vi "setup file.vi"(4 "frame rate":dbl, 5 "accel range":dbl, 6 "counts per rev":dbl, 7 "gyro range":dbl, 8 "error in (no error)":errorcluster, 11 "selected path":path) -> (0 "error out":errorcluster, 1 "channel names":string[](array[string]), 3 "tdms file out":refnum<k34>)   [LabVIEW 2012]
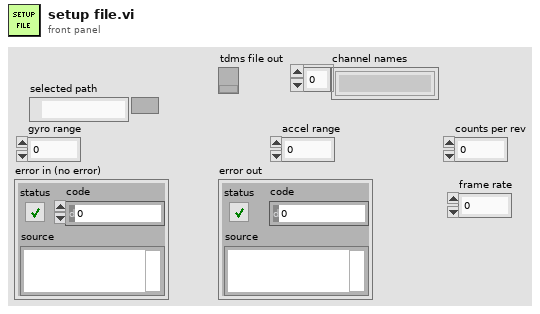
[diagram p1: front panel]
types:
  T1 = enum16{"open", "open or create", "create or replace", "create", "open (read-only)"}
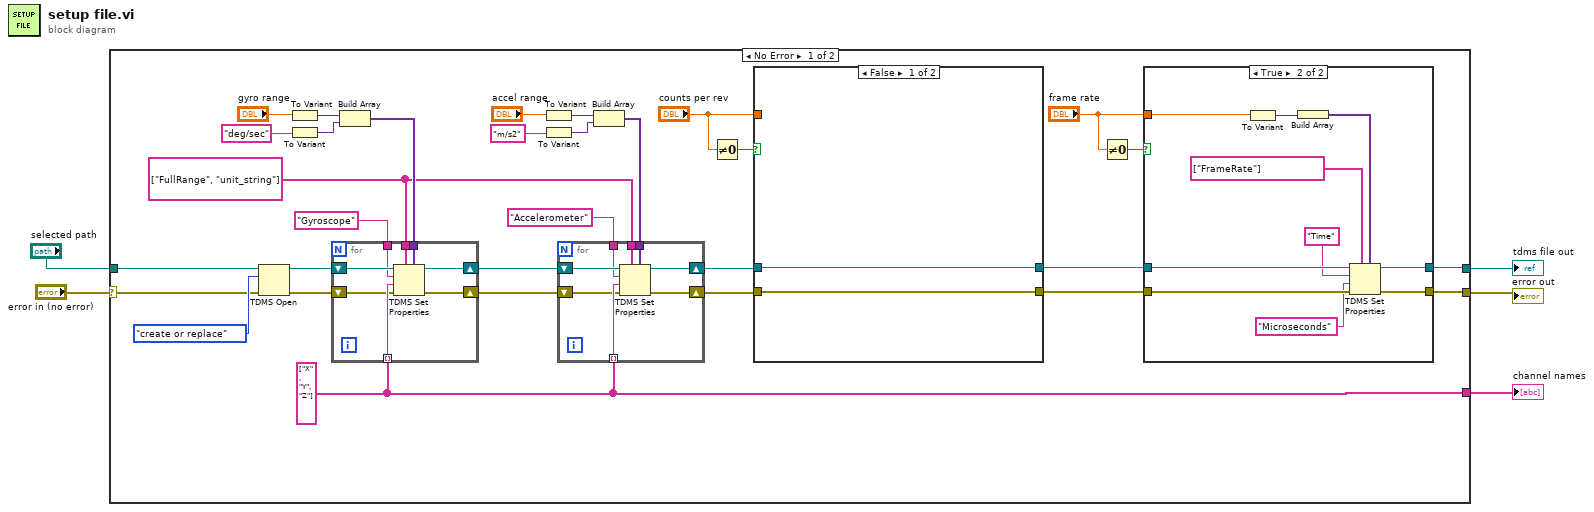
[diagram p0: block diagram]
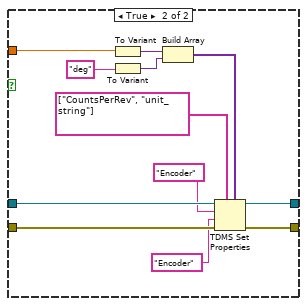
[diagram p3: hidden frame]
diagram:
  n1 = case shown="No Error" "error in (no error)" {
    selector: "error in (no error)" -> [w17 w79]
    tunnel: "selected path" -> [w35 _]
    tunnel: [w7 _] -> w3
    tunnel: [w6 w79] -> w2
    tunnel: [w16 _] -> w1
    frame No Error {
      w23 = string[] ["FullRange", "unit_string"] ("property names")
      w16 = string[] ["X", "Y", "Z"] ("channel name(s)")
      n2 = TDMS Open(8:w17, 10:T1."create or replace" ("operation (0:open)"), 11:w35) -> (0:w32:errorcluster, 3:w34:refnum<k34>)  [unwired: 3 in]
      n3 = To Variant(anything="gyro range") -> (Variant=w29:variant)
      n4 = To Variant(anything="deg/sec" ("group name (Untitled)")) -> (Variant=w28:variant)
      n5 = Build Array(w29, w28) -> (w27:variant[])
      n6 = for {
        tunnel: "Gyroscope" ("group name (Untitled)") -> [w77]
        tunnel: w16 -> [w76] mode=indexing
        shift-right: [w74] -> w24
        shift-left: w32 -> [w75]
        tunnel: w23 -> [w73]
        tunnel: w27 -> [w72]
        shift-right: [w71] -> w25
        shift-left: w34 -> [w78]
        n7 = TDMS Set Properties(5:w72, 7:w73, 8:w75, 9:w76, 10:w77, 11:w78) -> (0:w74:errorcluster, 3:w71:refnum<k34>)  [unwired: 2 out]
      }
      n8 = To Variant(anything="accel range") -> (Variant=w21:variant)
      n9 = To Variant(anything="m/s2" ("group name (Untitled)")) -> (Variant=w22:variant)
      n10 = Build Array(w21, w22) -> (w18:variant[])
      n11 = for {
        tunnel: "Accelerometer" ("group name (Untitled)") -> [w69]
        tunnel: w16 -> [w68] mode=indexing
        shift-right: [w66] -> w14
        shift-left: w24 -> [w67]
        tunnel: w23 -> [w65]
        tunnel: w18 -> [w64]
        shift-right: [w63] -> w15
        shift-left: w25 -> [w70]
        n12 = TDMS Set Properties(5:w64, 7:w65, 8:w67, 9:w68, 10:w69, 11:w70) -> (0:w66:errorcluster, 3:w63:refnum<k34>)  [unwired: 2 out]
      }
      n13 = Not Equal To 0?(x="counts per rev") -> (x != 0?=w12:bool)
      n14 = case shown="False" w12 {
        tunnel: w15 -> [w50 w62]
        tunnel: [w50 w61] -> w9
        tunnel: w14 -> [w49 w60]
        tunnel: [w49 w59] -> w8
        tunnel: "counts per rev" -> [_ w58]
        frame False {
        }
        frame True {
          n15 = To Variant(anything=w58) -> (Variant=w56:variant)
          n16 = To Variant(anything="deg" ("group name (Untitled)")) -> (Variant=w55:variant)
          n17 = Build Array(w56, w55) -> (w54:variant[])
          n18 = TDMS Set Properties(5:w54, 7:string[] ["CountsPerRev", "unit_string"] ("property names"), 8:w60, 9:"Encoder" ("group name"), 10:"Encoder" ("group name"), 11:w62) -> (0:w59:errorcluster, 3:w61:refnum<k34>)  [unwired: 2 out]
        }
      }
      n19 = Not Equal To 0?(x="frame rate") -> (x != 0?=w11:bool)
      n20 = case shown="True" w11 {
        tunnel: w9 -> [w38 w48]
        tunnel: [w38 w47] -> w7
        tunnel: w8 -> [w37 w46]
        tunnel: [w37 w45] -> w6
        tunnel: "frame rate" -> [_ w44]
        frame False {
        }
        frame True {
          n21 = To Variant(anything=w44) -> (Variant=w43:variant)
          n22 = Build Array(w43) -> (w42:variant[])
          n23 = TDMS Set Properties(5:w42, 7:string[] ["FrameRate"] ("property names"), 8:w46, 9:"Microseconds" ("group name"), 10:"Time" ("group name"), 11:w48) -> (0:w45:errorcluster, 3:w47:refnum<k34>)  [unwired: 2 out]
        }
      }
    }
    frame Error {
    }
  }
  "tdms file out" <- w3
  "error out" <- w2
  "channel names" <- w1
